vi "ROI_Image_Determine Circles.vi"(8 "error in (no error)":errorcluster, 11 "Image in":T1) -> (0 "error out":errorcluster, 1 "N Circles":i32, 2 "Biggest Circles Data":T2, 3 "Image out":T1)   [LabVIEW 2014]
uses:
  <vilib>/vision/Image Controls.llb/IMAQ Image.ctl
  FileIO/TypeDef - File Actions.ctl
  <vilib>/vision/NI_Vision_Development_Module.lvlib
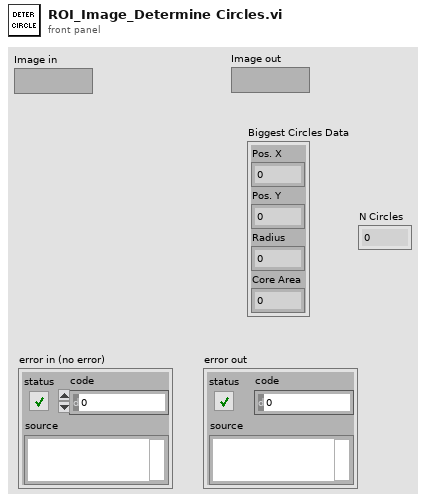
[diagram p1: front panel]
types:
  T1 = typedef "IMAQ Image.ctl" = refnum<image>
  T2 = cluster{"Pos. X":i32, "Pos. Y":i32, "Radius":i32, "Core Area":i32}
  T3 = typedef "TypeDef - File Actions.ctl" = enum16{"Read", "Write", "Get Current"}
  T4 = typedef "TypeDef - System Configuration.ctl" = cluster{"Results FilePath":path, "Analysis Parameters":cluster{"Area":cluster{"Lower Value":dbl, "Upper Value":dbl}, "Circle Filter Radius":cluster{"Lower Value":sgl, "Upper Value":sgl}, "Edge Detection Threshold":u16}, "ROI Parameters":cluster{"ROI size (in Radius)":cluster{"Width":dbl, "Height":dbl}}}
  T5 = cluster{"Pos. X":i32, "Pos. Y":i32, "Radius":i32, "Core Area":i32}[]
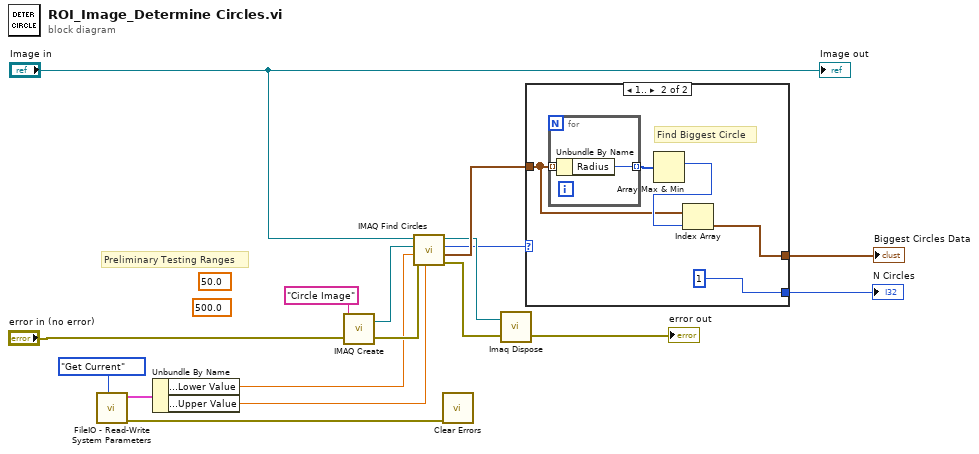
[diagram p0: block diagram]
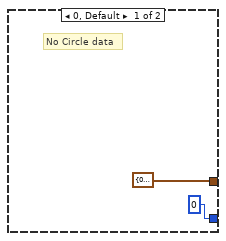
[diagram p2: hidden frame]
diagram:
  (unwired) sgl 500.0 ("Max Radius")
  (unwired) sgl 50.0 ("Min Radius")
  # "Preliminary Testing Ranges"
  n1 = call "FileIO - Read-Write System Parameters.vi"("Action"=TypeDef_-_File_Actions."Get Current") -> ("error out"=w7:errorcluster, "System Parameters out"=w8:T4)  [unwired: 9 in]
  n2 = Unbundle By Name(w8) -> ("Analysis Parameters.Circle Filter Radius.Lower Value"=w6:sgl, "Analysis Parameters.Circle Filter Radius.Upper Value"=w5:sgl)
  n3 = call "IMAQ Create"("Image Name"="Circle Image", "error in (no error)"="error in (no error)") -> ("New Image"=w16:T1, "error out"=w13:errorcluster)  [unwired: 2 in, 1 out]
  n4 = call "IMAQ Find Circles"("Max Radius"=w5, "error in (no error)"=w13, "Min Radius"=w6, "Image Dst"=w16, "Image Src"="Image in") -> ("error out"=w14:errorcluster, "Circles Data"=w12:T5, "Nb Circles"=w1:i32, "Image Dst Out"=w4:T1)  [unwired: 3 out]
  n5 = call <vilib>:"Clear Errors.vi"("error in (no error)"=w7) -> ()  [unwired: 5 in, 2 out]
  n6 = call "Imaq Dispose"("Image"=w4, "error in (no error)"=w14) -> ("error out"=→"error out":errorcluster)  [unwired: 4 in]
  n7 = case shown="1.." w1 {
    tunnel: w12 -> [_ w22]
    tunnel: [T2 {"Pos. X"=0, "Pos. Y"=0, "Radius"=0, "Core Area"=0} ("Circles Data") w21] -> w10
    tunnel: [0 1] -> w2
    frame 0, Default {
      # "No Circle data"
    }
    frame 1.. {
      # "Find Biggest Circle"
      n8 = for {
        tunnel: w22 -> [w26] mode=indexing
        tunnel: [w25] -> w23 mode=indexing
        n9 = Unbundle By Name(w26) -> ("Radius"=w25:i32)
      }
      n10 = Array Max & Min(array=w23) -> (max index (indices)=w24:i32)  [unwired: 3 out]
      n11 = Index Array(array=w22, index=w24) -> (element=w21:T2)
    }
  }
  "Biggest Circles Data" <- w10
  "N Circles" <- w2
  "Image out" <- "Image in"
